vi "MultiMFC.vi"() -> ()   [LabVIEW 2016]
panel:
  in  "Tab Control":enum32{"Page 1", "Page 2"}(tab)
  in  "Array":cluster{"Setpoint":dbl, "Valve":bool}[](array[cluster]) caption="Nitrogen       Nitrogen       Nitrogen       Nitrogen      Nitrogen         Ethane          Ethane          Ethane\n        100              100               100                30                   5                  0.3                  5                  30" {"Setpoint" max=100.0 step=10.0 scale=0.0..100.0}
  in  "Gas Release Cart":string
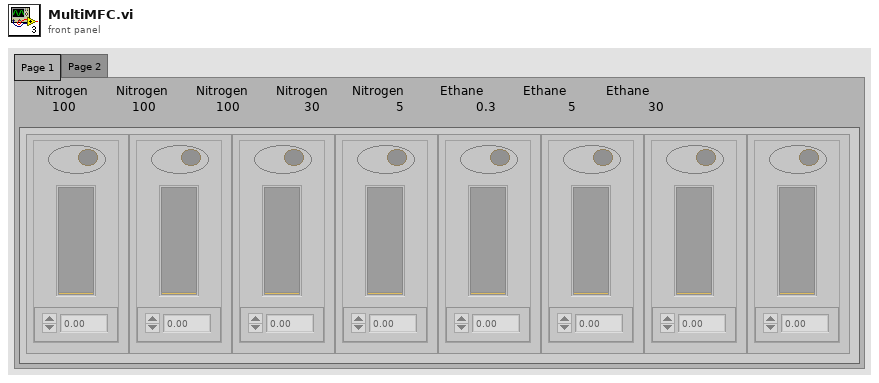
[diagram p1: front panel]
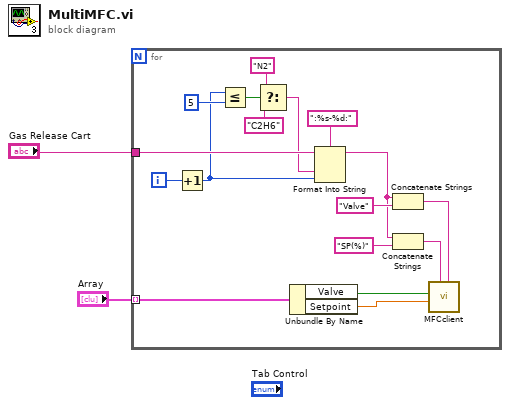
[diagram p0: block diagram]
diagram:
  n1 = for {
    tunnel: "Array" -> [w19] mode=indexing
    tunnel: "Gas Release Cart" -> [w8]
    i -> [w16]
    n2 = Increment(x=w16) -> (x+1=w6:i32)
    n3 = Less Or Equal?(x=w6, y=5) -> (x <= y?=w11:bool)
    n4 = Select(t="N2" ("string"), s=w11, f="C2H6" ("string")) -> (s? t:f=w5:string)
    n5 = Unbundle By Name(w19) -> ("Valve"=w18:bool, "Setpoint"=w17:dbl)
    n6 = Format Into String(format string=":%s-%d:", initial string=w8, w5, w6) -> (resulting string=w4:string)  [unwired: 1 in, 1 out]
    n7 = Concatenate Strings(w4, "Valve" ("string")) -> (w15:string)
    n8 = Concatenate Strings(w4, "SP(%)" ("string")) -> (w3:string)
    n9 = call "MFCclient.vi"("ValveName"=w15, "SPName"=w3, "Setpoint"=w17, "Valve"=w18) -> ()  [unwired: 8 in]
  }
